vi "INSERT (example).vi"() -> ()   [LabVIEW 2019, in "LV-Data.PGSQL.lvclass"]
uses:
  LV-Data.PGSQL.lvclass
panel:
  out "error out":errorcluster
  out "Wrote to DB?":bool
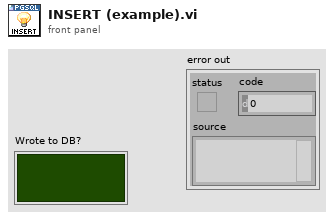
[diagram p1: front panel]
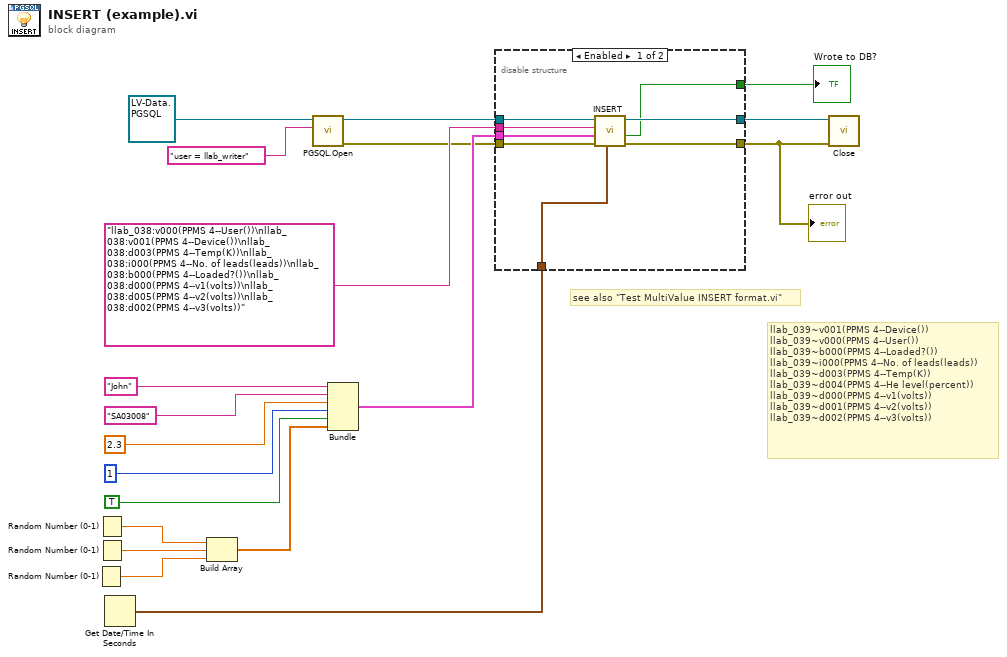
[diagram p0: block diagram]
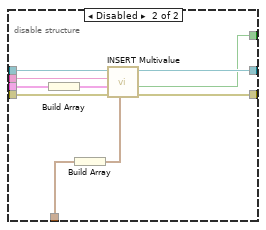
[diagram p2: hidden frame]
diagram:
  # "see also \"Test MultiValue INSERT format.vi\""
  # "llab_039~v001(PPMS 4--Device())\nllab_039~v000(PPMS 4--User())\nllab_039~b000(PPMS 4--Loaded?())\nllab_039~i000(PPMS 4--No. of leads(leads))\nllab_039~d003(PPMS 4--Temp(K))\nllab_039~d004(PPMS 4--He level(percent))\nllab_039~d000(PPMS 4--v1(volts))\nllab_039~d001(PPMS 4--v2(volts))\nllab_039~d002(PPMS 4--v3(volts))"
  n1 = Random Number (0-1)() -> (number: 0 to 1=w10:dbl)
  n2 = Random Number (0-1)() -> (number: 0 to 1=w8:dbl)
  n3 = Random Number (0-1)() -> (number: 0 to 1=w9:dbl)
  n4 = Get Date/Time In Seconds() -> (seconds since 1Jan1904=w17:timestamp)
  n5 = Build Array(w8, w9, w10) -> (w12:dbl[])
  n6 = call "PGSQL.Open.vi"("Connection String"="user = llab_writer", "Data.PG in"=refnum<class "LV-Data.PGSQL.lvclass"> refnum) -> ("error out"=w3:errorcluster, "Data.PG out"=w5:refnum<class "LV-Data.PGSQL.lvclass">)  [unwired: 8 in]
  n7 = Bundle("John", "SA03008", 2.3, 1, TRUE, w12) -> (w19:cluster{string, string, dbl, i32, bool, dbl[]})  [unwired: 1 in]
  n8 = disable-structure shown="Enabled" {
    disable-tunnel: w19 -> [w27 w30]
    disable-tunnel: "llab_038:v000(PPMS 4--User())\nllab_038:v001(PPMS 4--Device())\nllab_038:d003(PPMS 4--Temp(K))\nllab_038:i000(PPMS 4--No. of leads(leads))\nllab_038:b000(PPMS 4--Loaded?())\nllab_038:d000(PPMS 4--v1(volts))\nllab_038:d005(PPMS 4--v2(volts))\nllab_038:d002(PPMS 4--v3(volts))" -> [w26 w37]
    disable-tunnel: w17 -> [w25 w28]
    disable-tunnel: [w24 w36] -> w7
    disable-tunnel: w5 -> [w23 w35]
    disable-tunnel: w3 -> [w22 w34]
    disable-tunnel: [w21 w33] -> w2
    disable-tunnel: [w20 w32] -> w1
    frame Enabled {
      n9 = call "INSERT.vi"("Time Stamp"=w25, "error in"=w22, "Data"=w27, "Path(s)"=w26, "Data.PG in"=w23) -> ("error out"=w21:errorcluster, "Wrote to DB?"=w20:bool, "Data.PG out"=w24:refnum<class "LV-Data.PGSQL.lvclass">)  [unwired: 3 in, 1 out]
    }
    frame Disabled {
      n10 = Build Array(w30) -> (w31:cluster{string, string, dbl, i32, bool, dbl[]}[])
      n11 = Build Array(w28) -> (w29:timestamp[])
      n12 = call "INSERT Multivalue.vi"("Array"=w29, "error in"=w34, "Data"=w31, "Path(s)"=w37, "Data.PG in"=w35) -> ("error out"=w33:errorcluster, "Wrote All to DB?"=w32:bool, "Data.PG out"=w36:refnum<class "LV-Data.PGSQL.lvclass">)  [unwired: 3 in, 1 out]
    }
  }
  "Wrote to DB?" <- w1
  "error out" <- w2
  n13 = call-dynamic "Close.vi"("error in (no error)"=w2, "Data.PG in"=w7) -> ()  [unwired: 8 in, 2 out]
